vi "Apply Weights.vi"(0 "Noise in":refnum<class "Noise.lvclass">, 7 "Fs (Hz)":dbl, 9 "Npts":i32, 11 "error in (no error)":errorcluster) -> (4 "Noise out":refnum<class "Noise.lvclass">, 8 "noise":dbl[](array[numeric]), 10 "reference":dbl, 15 "error out":errorcluster)   [LabVIEW 2020, in "Noise.lvclass"]
uses:
  Noise.lvclass
  Noise.lvclass/Noise.ctl
  f3eec849-1a7e-4540-b510-488890d9b2c3.vi
  cf240ed5-2244-4fd4-95da-4ca8c54e370a.vi
  b45a6538-8973-4492-8a39-eff9211a81fe.vi
  Utility VIs/Math VIs/FFT x(t) to dB,Degrees (1D).vi
  <vilib>/Analysis/NI_AALBase.lvlib
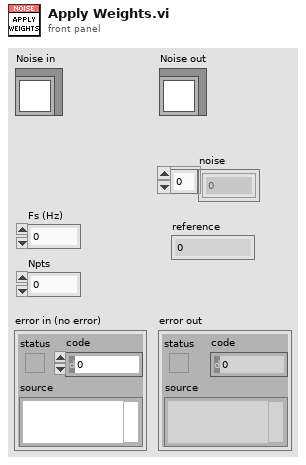
[diagram p1: front panel]
types:
  T1 = typedef "Noise.lvclass/Weighting.ctl" = enum16{"White", "Pink"}
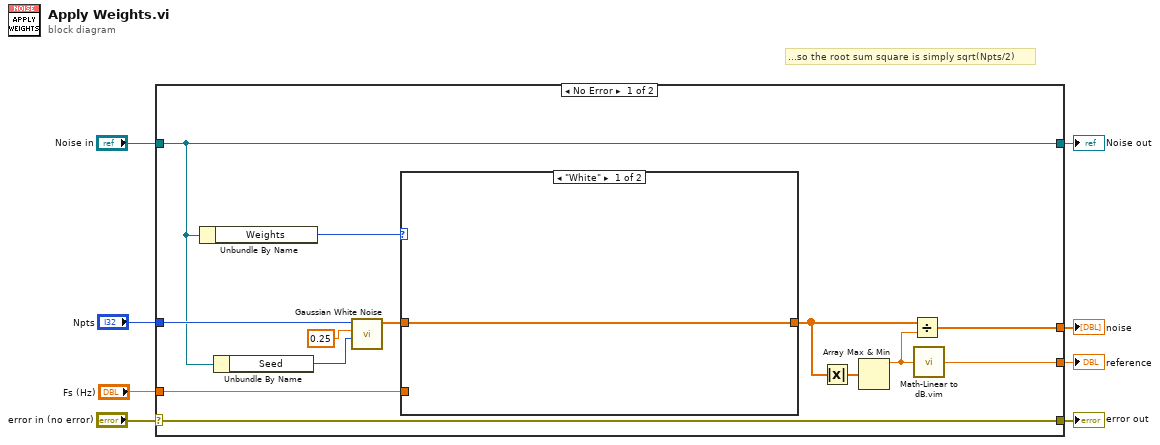
[diagram p0: block diagram]
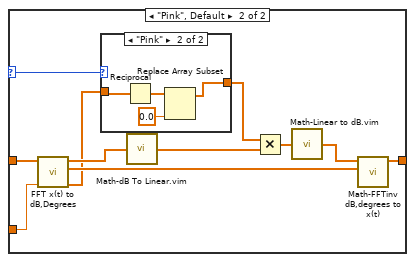
[diagram p2: hidden frame]
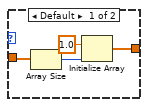
[diagram p3: hidden frame]
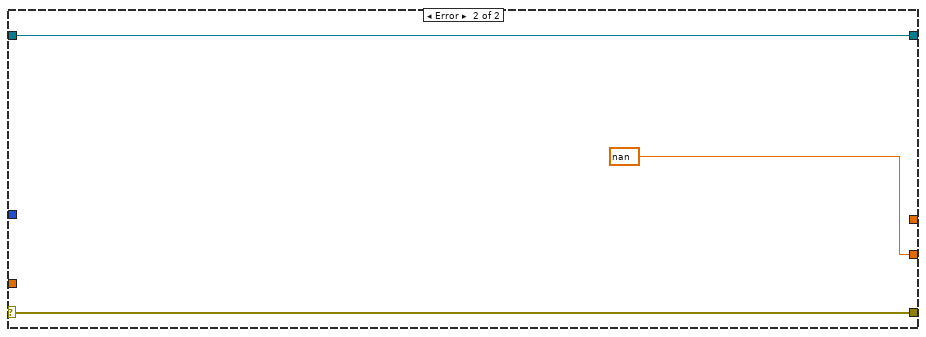
[diagram p4: hidden frame]
diagram:
  # "...so the root sum square is simply sqrt(Npts/2)"
  n1 = case shown="No Error" "error in (no error)" {
    selector: "error in (no error)" -> [w21 w44]
    tunnel: [w21 w44] -> w7
    tunnel: [w12 w43] -> w5
    tunnel: "Noise in" -> [w12 w43]
    tunnel: "Npts" -> [w13 _]
    tunnel: "Fs (Hz)" -> [w11 _]
    tunnel: [w9 nan] -> w2
    tunnel: [w15 _] -> w1
    frame No Error {
      n2 = Unbundle By Name(w12) -> ("Weights"=w10:T1)
      n3 = Unbundle By Name(w12) -> ("Seed"=w19:i32)
      n4 = call <vilib>:"Gaussian White Noise.vi"("seed"=w19, "standard deviation"=0.25, "samples"=w13) -> ("Gaussian noise pattern"=w18:dbl[])  [unwired: 7 in, 1 out]
      n5 = case shown="\"White\"" w10 {
        selector: w10 -> [_ w28]
        tunnel: w18 -> [w22 w33]
        tunnel: [w22 w31] -> w14
        tunnel: w11 -> [_ w30]
        frame "White" {
        }
        frame "Pink", Default {
          n6 = call-poly "FFT x(t) to dB,Degrees.vi"("Fs (Hz)"=w30, "X"=w33) -> ("Freq (Hz)"=w27:dbl[], "+Freq Phase of FFT (degrees)"=w32:dbl[], "+Freq. Mag of FFT (dB rms)"=w29:dbl[])  [unwired: 7 in]
          n7 = case shown="\"Pink\"" w28 {
            tunnel: w27 -> [w37 w41]
            tunnel: [w34 w38] -> w25
            frame Default {
              n8 = Array Size(array=w37) -> (size(s)=w36:i32)
              n9 = Initialize Array(1.0 ("element"), w36) -> (w34:dbl[])
            }
            frame "Pink" {
              n10 = Reciprocal(x=w41) -> (1/x=w40:dbl[])
              n11 = Replace Array Subset(array=w40, new element=0.0 ("new element/subarray")) -> (w38:dbl[])  [unwired: 1 in]
            }
          }
          n12 = call "Math-dB To Linear.vim"("dB"=w29) -> ("linear"=w26:dbl[])
          n13 = Multiply(x=w25, y=w26) -> (x*y=w24:dbl[])
          n14 = call "Math-Linear to dB.vim"("linear"=w24) -> ("dB"=w23:dbl[])
          n15 = call "Math-FFTinv dB,degrees to x(t).vi"("+Freq Phase of FFT (degrees)"=w32, "+Freq. Mag of FFT (rms dB)"=w23) -> ("X(t)"=w31:dbl[])  [unwired: 8 in, 1 out]
        }
      }
      n16 = Absolute Value(x=w14) -> (abs(x)=w17:dbl[])
      n17 = Array Max & Min(array=w17) -> (max value=w16:dbl)  [unwired: 3 out]
      n18 = Divide(x=w14, y=w16) -> (x/y=w15:dbl[])
      n19 = call "Math-Linear to dB.vim"("linear"=w16) -> ("dB"=w9:dbl)
    }
    frame Error {
    }
  }
  "error out" <- w7
  "Noise out" <- w5
  "reference" <- w2
  "noise" <- w1
